vi "Get Grid Marker.vi"(8 "Error In":errorcluster) -> (0 "error out":errorcluster, 3 "GMarker":refnum<k24>)   [LabVIEW 2014]
uses:
  C:/Robotic Systems/Products/AgFalcon/Software/Ground Station/Data/Mapping DLL/GMap.NET.WindowsForms.dll
  Data/Mapping DLL/GMap.NET.WindowsForms.dll
  Lat Long Conversion/Controls/PointLatLon.ctl
  C:/Robotic Systems/Products/AgFalcon/Software/Ground Station/Data/Mapping DLL/GMap.NET.Core.dll
  Data/Mapping DLL/GMap.NET.Core.dll
panel:
  in  "Origin Point":T1 {"Latitude" format="%#_10g"; "Longitude" format="%#_10g"}
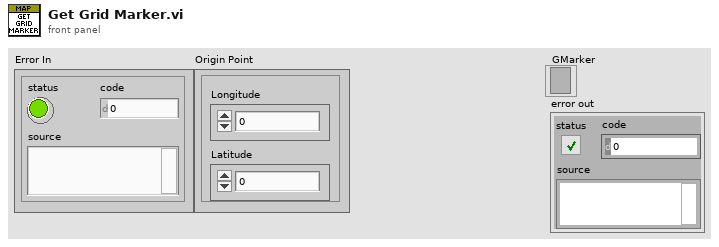
[diagram p1: front panel]
types:
  T1 = typedef "PointLatLon.ctl" = cluster{"Longitude":dbl, "Latitude":dbl}
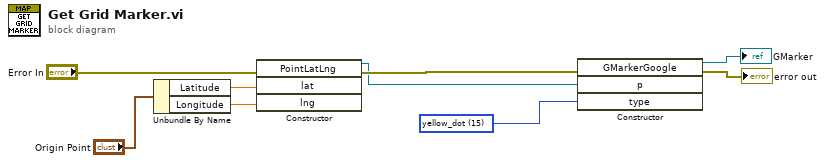
[diagram p0: block diagram]
diagram:
  w1 = 15 items=["none", "arrow", "blue", "blue_small", "blue_dot", "blue_pushpin", "brown_small", "gray_small", "green", "green_small", "green_dot", "green_pushpin", "green_big_go", "yellow", "yellow_small", "yellow_dot", "yellow_big_pause", "yellow_pushpin", "lightblue", "lightblue_dot", "lightblue_pushpin", "orange", "orange_small", "orange_dot", "pink", "pink_dot", "pink_pushpin", "purple", "purple_small", "purple_dot", "purple_pushpin", "red", "red_small", "red_dot", "red_pushpin", "red_big_stop", "black_small", "white_small"] ("type")
  n1 = Unbundle By Name("Origin Point") -> ("Latitude"=w4:dbl, "Longitude"=w3:dbl)
  n2 = constructor class="PointLatLng"(error in="Error In", "lat"=w4, "lng"=w3) -> (reference out=w2:refnum<k24>, error out=w6:errorcluster)  [unwired: 2 in, 3 out]
  n3 = constructor class="GMarkerGoogle"(error in=w6, "p"=w2, "type"=w1) -> (reference out=→"GMarker":refnum<k24>, error out=→"error out":errorcluster)  [unwired: 2 in, 3 out]
